vi "Updateinter.vi"(10 "更新包远端地址":string="/updatefiles/OneStation/V4/一体化微型水质监测站.zip", 11 "测试版？":bool) -> ()   [LabVIEW 2016, in "数据传输系统.lvlib" / "update.lvlib"]
uses:
  update.lvlib
  <vilib>/Utility/miscctls.llb/LVPointTypeDef.ctl
  WebDAV client/WebDAV client.lvclass
panel:
  out "已下载大小":sgl format="%.2f MB"
  out "滑动杆":dbl(slide) scale=0.0..100.0
  in  "取消按钮":bool
  out "last status string":string caption="最近状态字符串"
  out "command":string caption="命令"
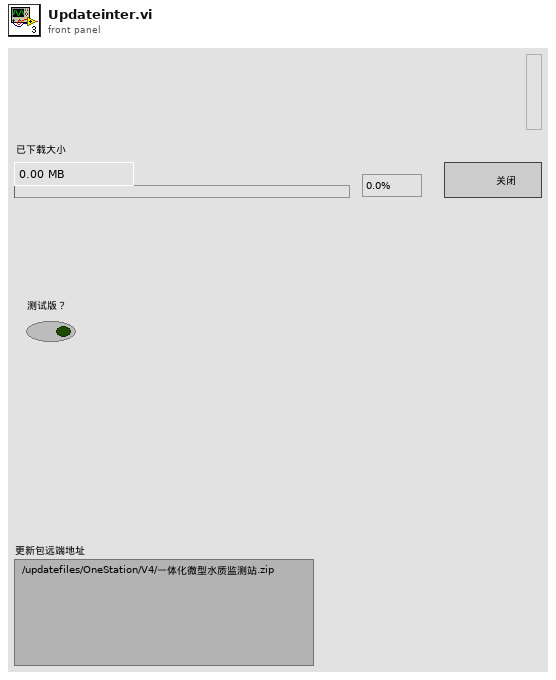
[diagram p1: front panel]
types:
  T1 = typedef "LVPointTypeDef.ctl" = cluster{"Horizontal":i16, "Vertical":i16}
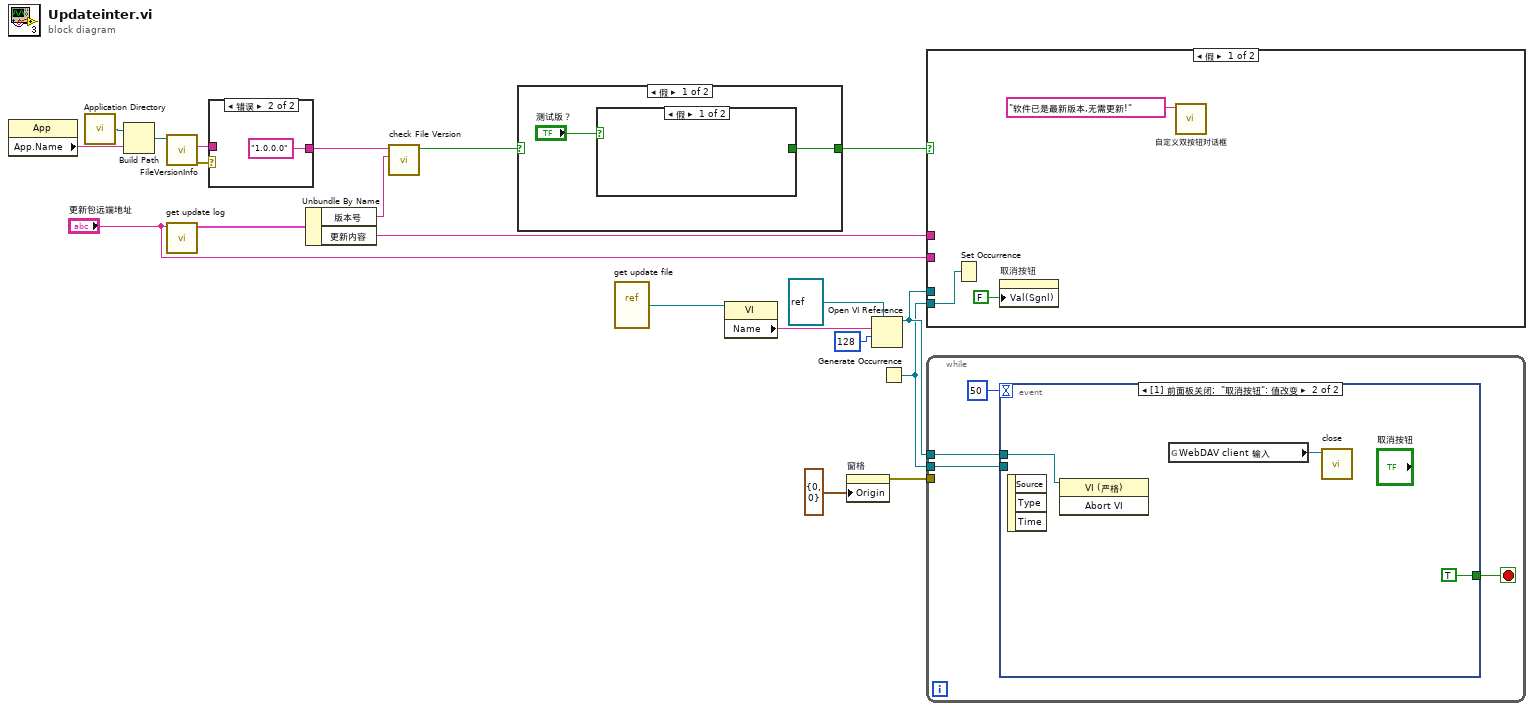
[diagram p0: block diagram]
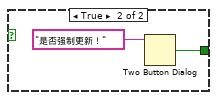
[diagram p3: hidden frame]
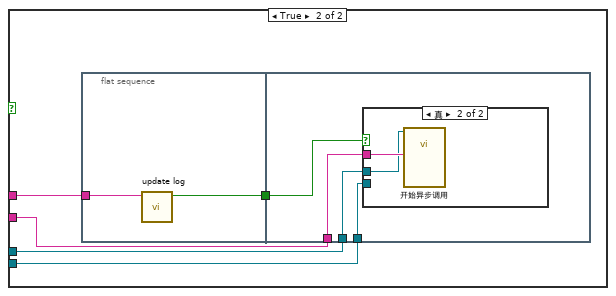
[diagram p5: hidden frame]
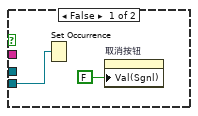
[diagram p6: hidden frame]
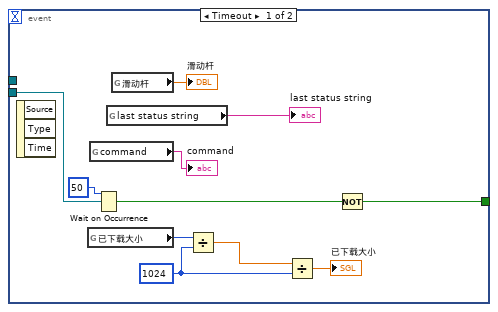
[diagram p7: hidden frame]
diagram:
  n1 = property class="App"() -> ("App.Name"=w20:string)  [unwired: 2 in, 2 out]
  n2 = call <vilib>:"Application Directory.vi"() -> ("Application Directory"=w13:path)
  n3 = Build Path(base path=w13, name or relative path=w20) -> (appended path=w19:path)
  n4 = call <vilib>:"FileVersionInfo.vi"("Application Path in"=w19) -> ("error out"=w3:errorcluster, "File Version Info"=w2:string)  [unwired: 7 in, 2 out]
  n5 = call "get update log.vi"("远端地址"="更新包远端地址") -> ("元素"=w14:cluster{"版本号":string, "更新内容":string})  [unwired: 8 in, 2 out]
  n6 = case shown="错误" w3 {
    tunnel: [w21 "1.0.0.0" ("File Version Info")] -> w1
    tunnel: w2 -> [w21 _]
    frame No Error {
    }
    frame Error {
    }
  }
  n7 = Unbundle By Name(w14) -> ("版本号"=w12:string, "更新内容"=w11:string)
  n8 = call "check File Version.vi"("remote File Version Info"=w12, "Local File Version Info"=w1) -> ("new?"=w18:bool)  [unwired: 9 in]
  n9 = case shown="假" w18 {
    selector: w18 -> [_ w27]
    tunnel: [w23 w27] -> w17
    frame False {
      n10 = case shown="假" "测试版？" {
        tunnel: [_ w26] -> w23
        frame False {
        }
        frame True {
          n11 = Two Button Dialog(message="是否强制更新！" ("消息")) -> (T button?=w26:bool)  [unwired: 2 in]
        }
      }
    }
    frame True {
    }
  }
  n12 = vi-ref "get update file.vi"() -> (w7:refnum<vi>)
  n13 = property class="VI"(reference=w7) -> ("Name"=w8:string)  [unwired: 1 in, 2 out]
  n14 = property on="窗格" class="Pane"("Origin"=T1 {"Horizontal"=0, "Vertical"=0} ("原点")) -> (error out=w16:errorcluster)  [unwired: 2 in, 1 out]
  n15 = Open VI Reference(type specifier VI Refnum (for type only)=refnum<vi> refnum, vi path=w8, options=128 ("选项")) -> (vi reference=w6:refnum<vi>)  [unwired: 3 in, 1 out]
  n16 = Generate Occurrence() -> (w5:refnum<k4>)
  n17 = case shown="假" w17 {
    tunnel: w11 -> [_ w35]
    tunnel: "更新包远端地址" -> [_ w33]
    tunnel: w6 -> [_ w32]
    tunnel: w5 -> [w29 w31]
    frame False {
      n18 = Set Occurrence(w29) -> ()
      n19 = property on="取消按钮" class="Bool (严格)"("Val(Sgnl)"=FALSE ("值(信号)")) -> ()  [unwired: 2 in, 2 out]
      n20 = call "自定义双按钮对话框.vi"("消息"="软件已是最新版本,无需更新!") -> ()  [unwired: 10 in, 1 out]
    }
    frame True {
      n21 = flat-sequence {
        tunnel: w35 -> [w37]
        tunnel: [w36] -> w34
        tunnel: w34 -> [w41]
        tunnel: w33 -> [w40]
        tunnel: w32 -> [w39]
        tunnel: w31 -> [w38]
        frame #0 {
          n22 = call "update log.vi"("更新记录"=w37) -> ("check"=w36:bool)  [unwired: 10 in]
        }
        frame #1 {
          n23 = case shown="真" w41 {
            tunnel: w40 -> [_ w45]
            tunnel: w39 -> [_ w44]
            tunnel: w38 -> [w43 _]
            frame False {
              n24 = Set Occurrence(w43) -> ()
              n25 = property on="取消按钮" class="Bool (严格)"("Val(Sgnl)"=FALSE ("值(信号)")) -> ()  [unwired: 2 in, 2 out]
            }
            frame True {
              n26 = call-by-ref "开始异步调用"(reference=w44, "远端地址"=w45) -> ()  [unwired: 11 in, 3 out]
            }
          }
        }
      }
    }
  }
  n27 = while {
    tunnel: w16 -> [_]
    tunnel: w6 -> [w47]
    tunnel: w5 -> [w46]
    stop <- w48 stop-if-true
    n28 = event shown="[1] 前面板关闭;  \"取消按钮\": 值改变" {
      selector: _ -> [_ _]
      dyn-events: _ -> [_ _]
      timeout: 50 -> [_ _]
      tunnel: [w50 TRUE] -> w48
      tunnel: w47 -> [_ w62]
      tunnel: w46 -> [w55 _]
      event Timeout {
        w56 = i64 1024 ("y")
        n29 = event-data() -> ()  [unwired: 1 in, 3 out]
        n30 = global read "更新全局变量.vi" "已下载大小"() -> (w58:i64)
        n31 = global read "更新全局变量.vi" "command"() -> (→"command":string)
        n32 = Wait on Occurrence(2:w55, 3:50 ("毫秒超时(-1)")) -> (0:w53:bool)  [unwired: 1 in]
        n33 = global read "更新全局变量.vi" "last status string"() -> (→"last status string":string)
        n34 = global read "更新全局变量.vi" "滑动杆"() -> (→"滑动杆":dbl)
        n35 = Divide(x=w58, y=w56) -> (x/y=w57:dbl)
        n36 = Divide(x=w57, y=w56) -> (x/y=→"已下载大小":dbl)
        n37 = Not(x=w53) -> (.not. x?=w50:bool)
      }
      event Panel Close; "取消按钮": Value Change {
        n38 = event-data() -> ()  [unwired: 1 in, 3 out]
        n39 = invoke class="VI (严格)" method="Abort VI"(reference=w62) -> ()  [unwired: 2 in, 3 out]
        n40 = global read "更新全局变量.vi" "WebDAV client 输入"() -> (w61:refnum<class "WebDAV client.lvclass">)
        n41 = call-dynamic "close.vi"("WebDAV client 输入"=w61) -> ()  [unwired: 9 in, 2 out]
      }
    }
  }
